vi "map_trap_switch_stiffback.vi"() -> ()   [LabVIEW 2015]
panel:
  out "Mapping file":string
  in  "Done ?":bool
  in  "KILL":bool
  in  "PAUSE":bool
  in  "RESUME":bool
  in  "QUIT":bool
  in  "up done":bool
  in  "z up":bool
  in  "Done":bool
  in  "z piastra":bool
  in  "x piastra":bool
  in  "goto y pos":bool
  in  "goto x pos":bool
  in  "End":bool
  in  "zero z - end":bool
  in  "zero x - end":bool
  in  "zero y - end":bool
  in  "positioning done":bool
  out "output":string
  out "command":string
  in  "zero done":bool
  in  "zero z":bool
  in  "zero x":bool
  in  "zero y":bool
  # "Comandi di emergenza"
  # "Posiziono in zero"
  # "Vado sulla piastra \ne azzero"
  # "Alzo il laser"
  # "Vado in posizione"
  # "Ritorno a zero"
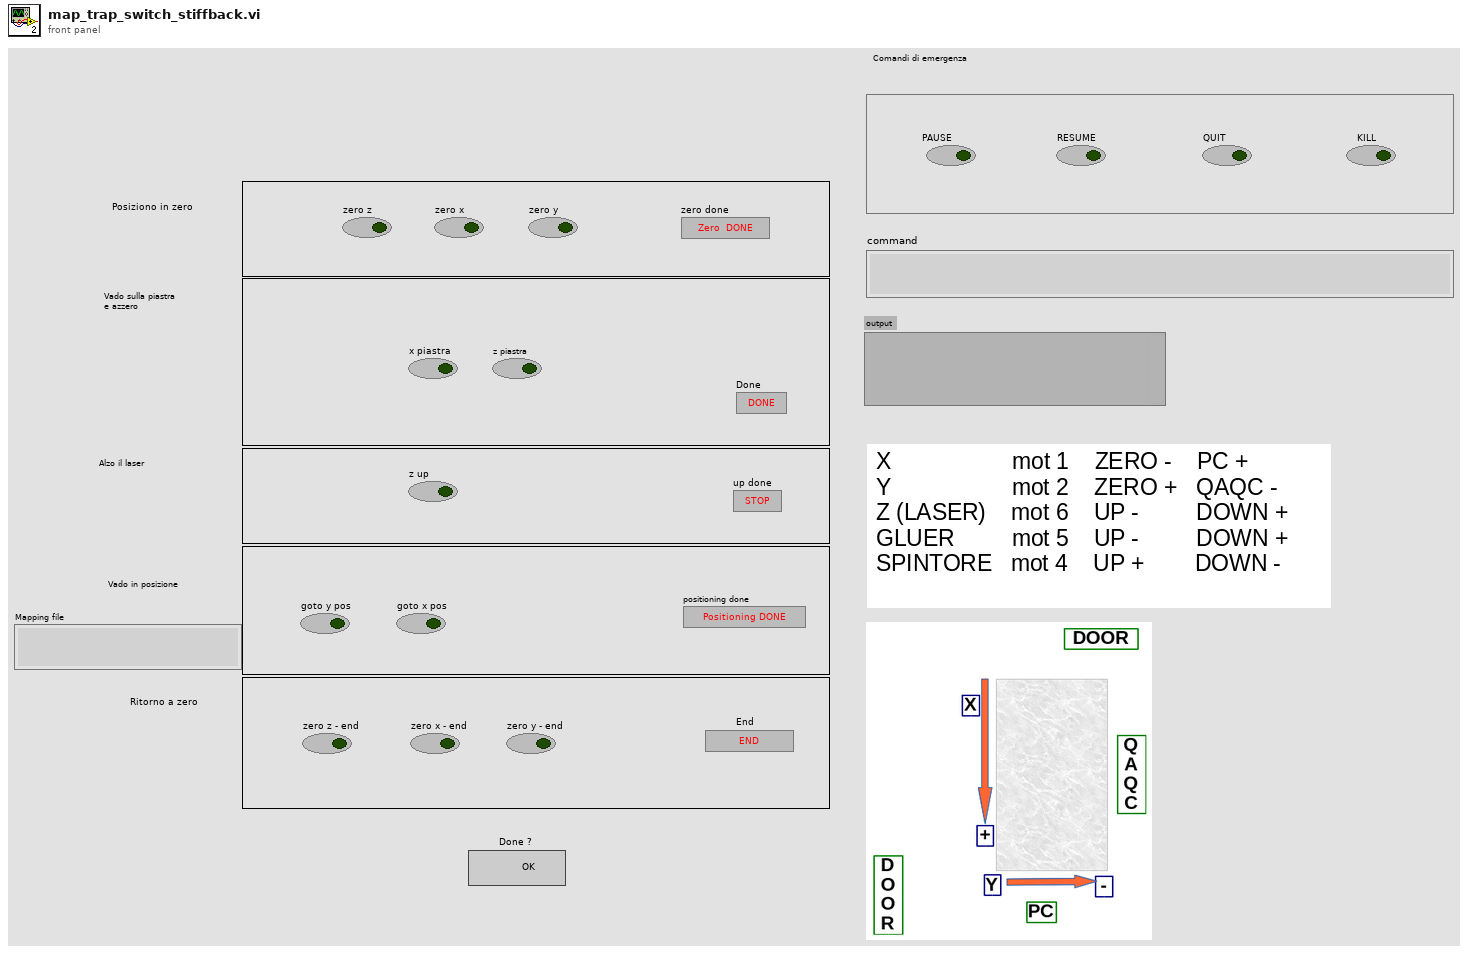
[diagram p1: front panel]
types:
  T1 = enum16{"open", "replace", "create", "open or create", "replace or create", "replace or create with confirmation"}
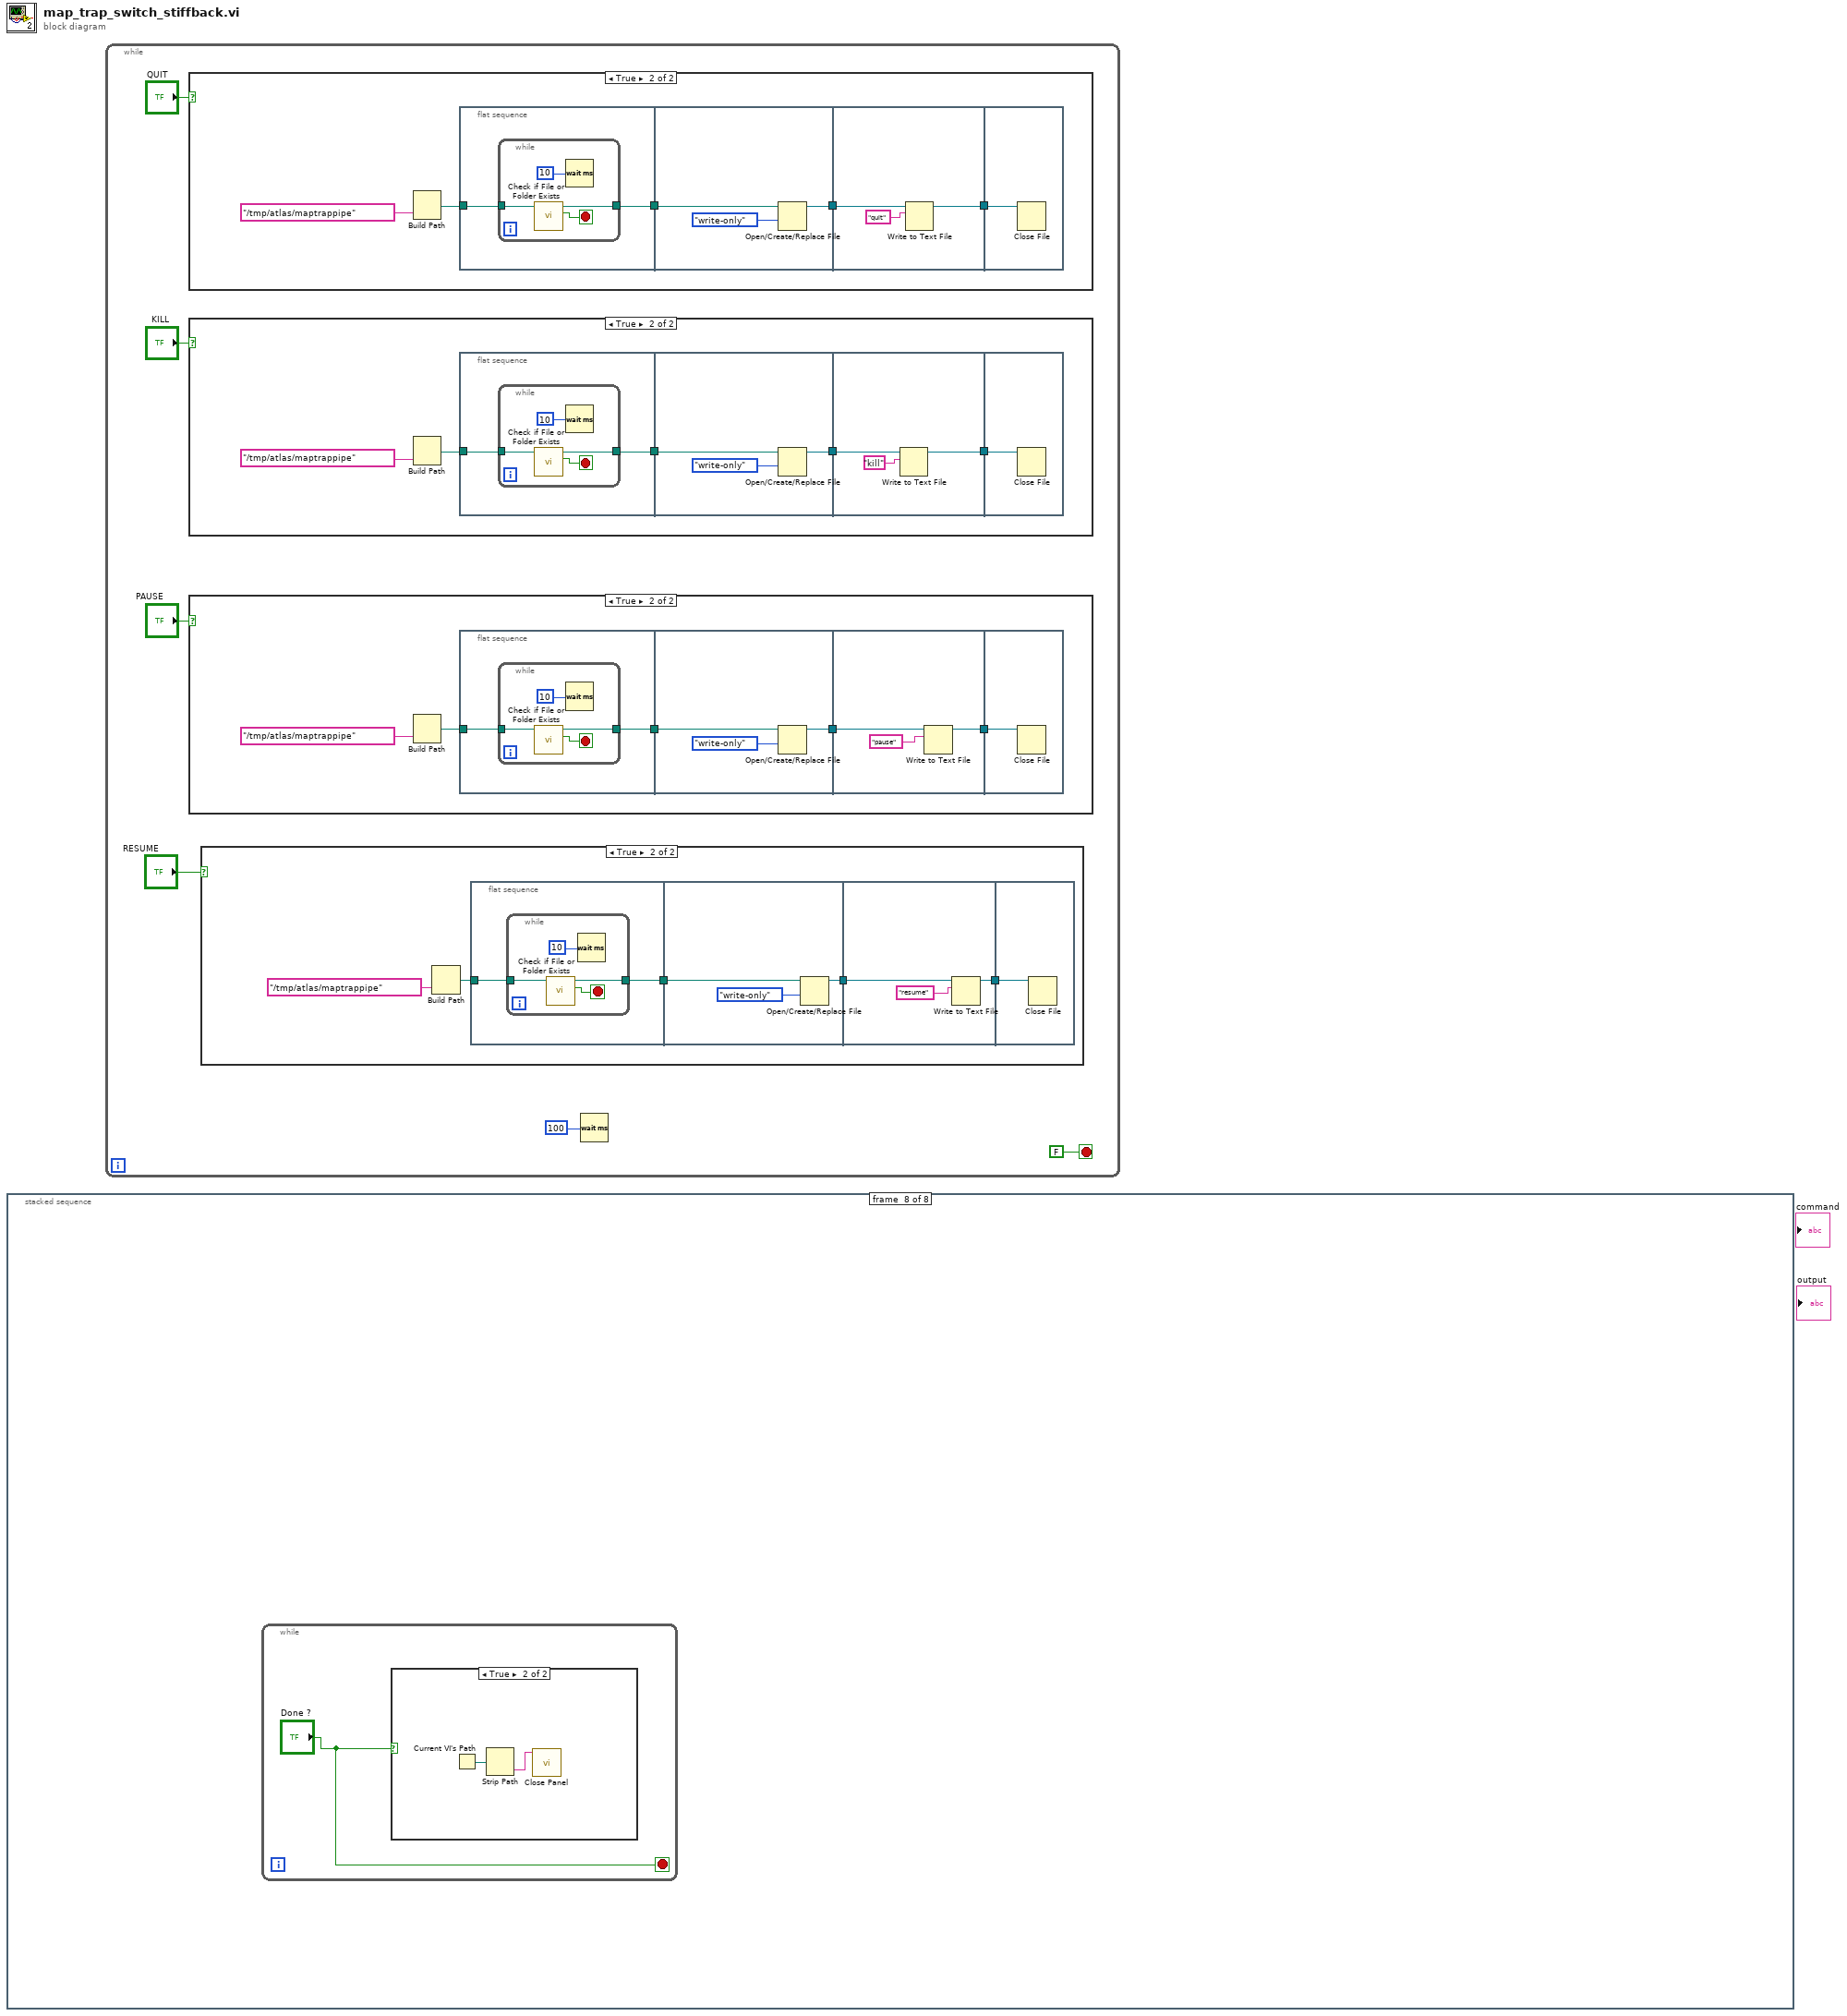
[diagram p0: block diagram]
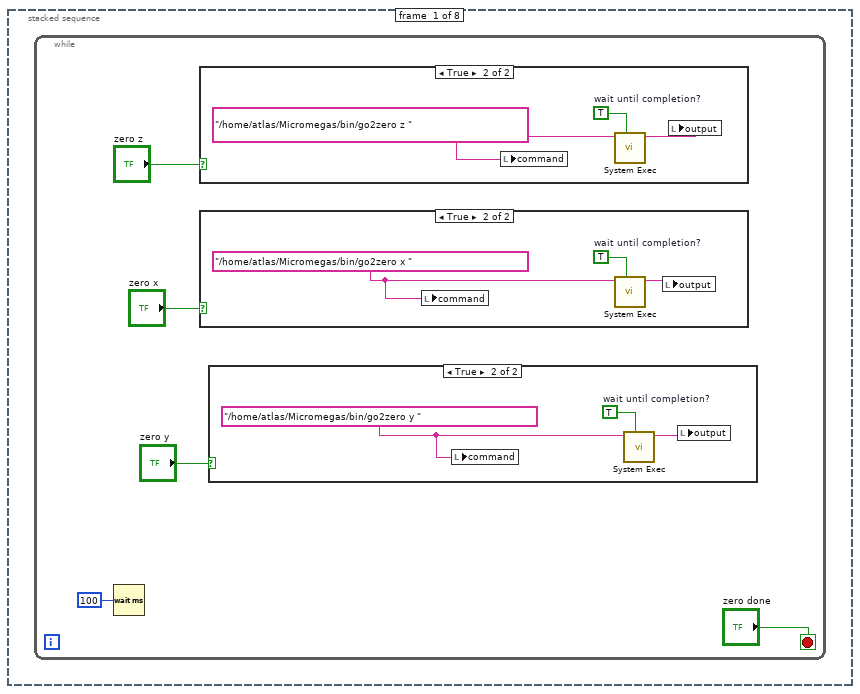
[diagram p6: hidden frame]
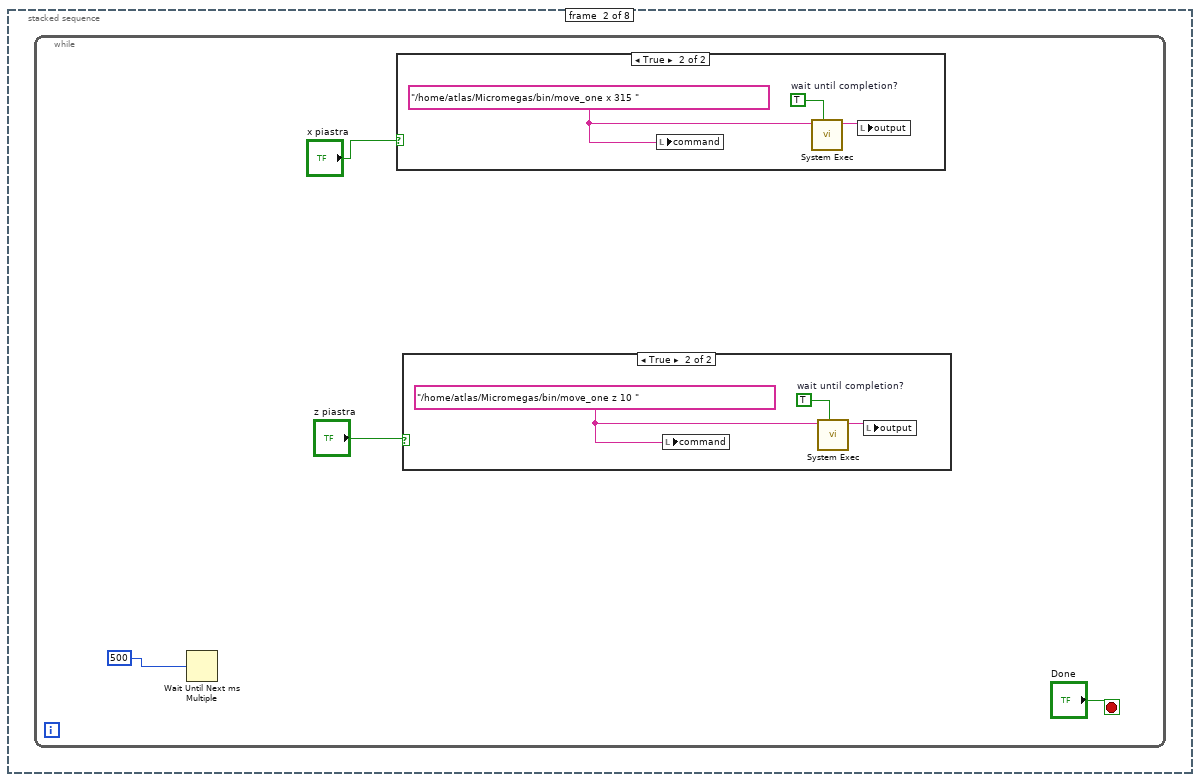
[diagram p10: hidden frame]
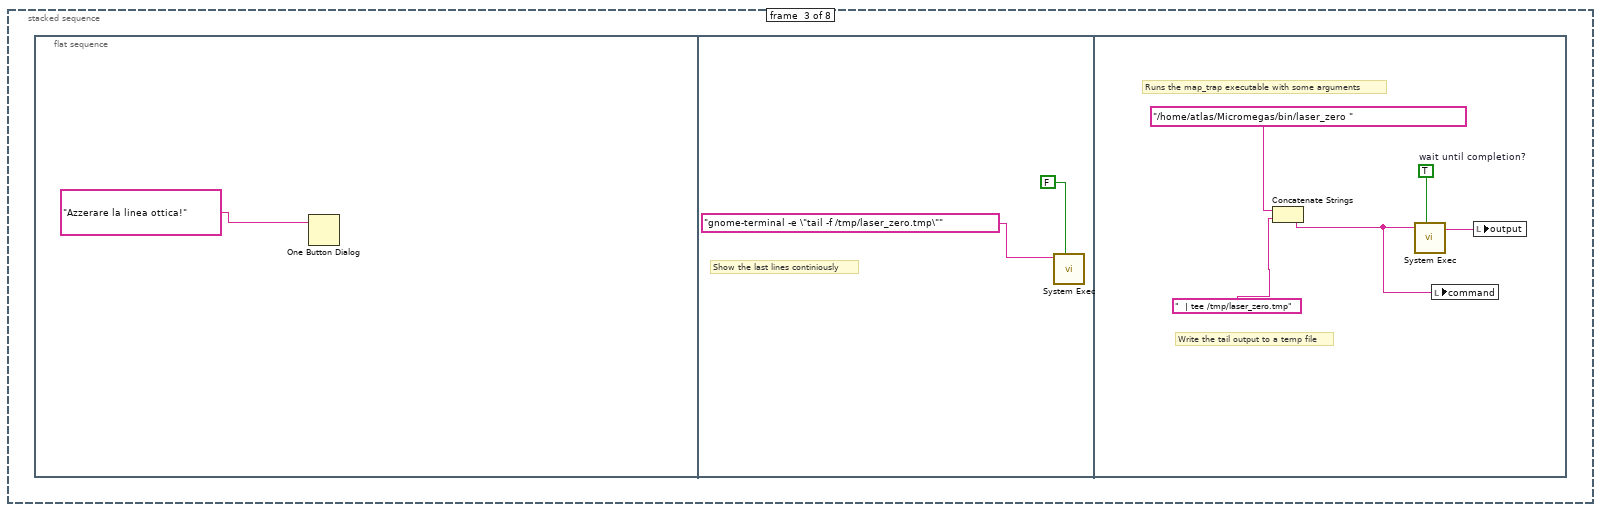
[diagram p13: hidden frame]
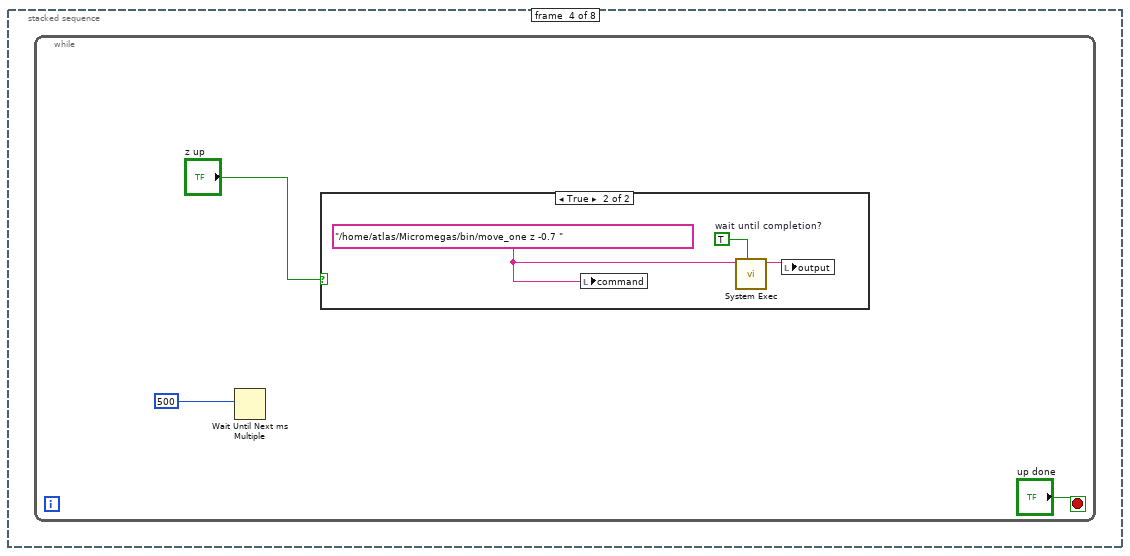
[diagram p14: hidden frame]
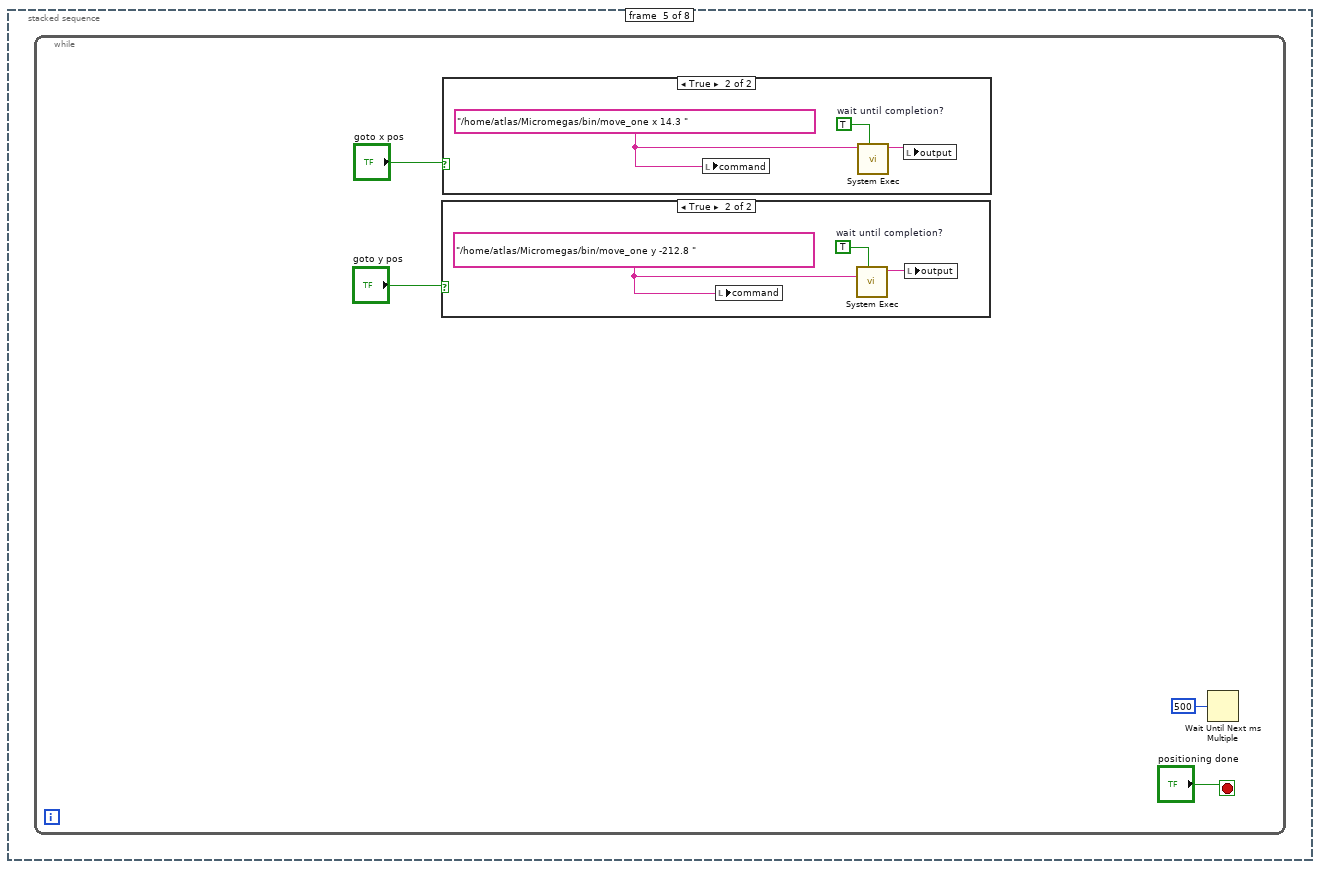
[diagram p16: hidden frame]
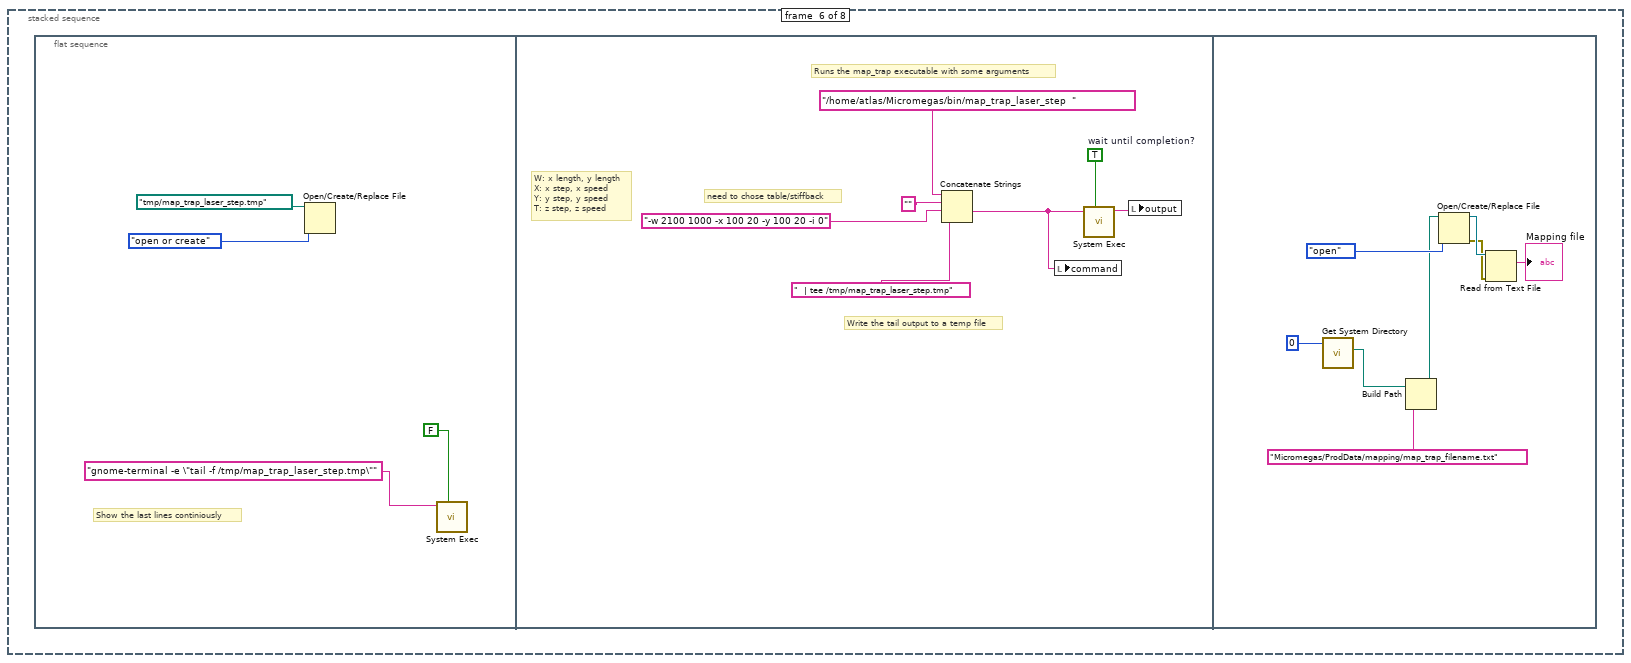
[diagram p19: hidden frame]
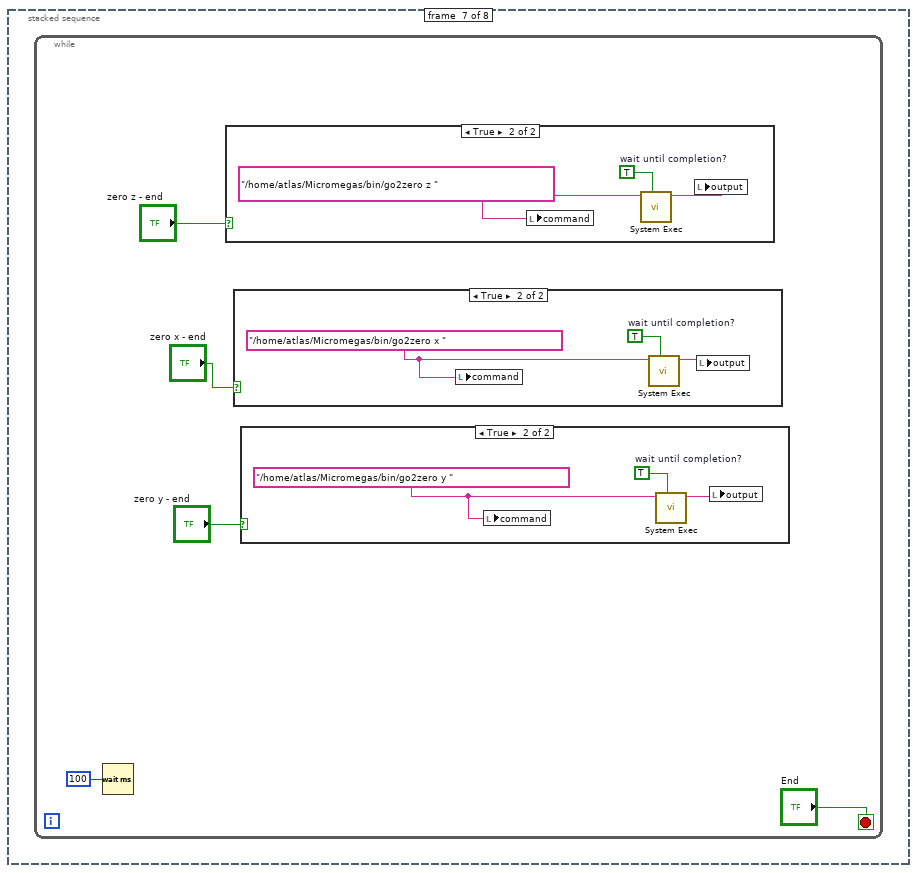
[diagram p20: hidden frame]
diagram:
  n1 = stacked-sequence {
    frame #0 {
      n2 = while {
        stop <- "zero done" stop-if-true
        n3 = Wait (ms)(milliseconds to wait=u32 100) -> ()  [unwired: 1 out]
        n4 = case shown="True" "zero z" {
          frame False {
          }
          frame True {
            w13 = "/home/atlas/Micromegas/bin/go2zero z " ("string")
            w14 = TRUE  # wait until completion?
            n5 = local write "command"(w13) -> ()
            n6 = call <vilib>:"System Exec.vi"("wait until completion? (T)"=w14, "command line"=w13) -> ("standard output"=w12:string)  [unwired: 6 in, 3 out]
            n7 = local write "output"(w12) -> ()
          }
        }
        n8 = case shown="True" "zero x" {
          frame False {
          }
          frame True {
            w10 = "/home/atlas/Micromegas/bin/go2zero x " ("string")
            w11 = TRUE  # wait until completion?
            n9 = local write "command"(w10) -> ()
            n10 = call <vilib>:"System Exec.vi"("wait until completion? (T)"=w11, "command line"=w10) -> ("standard output"=w9:string)  [unwired: 6 in, 3 out]
            n11 = local write "output"(w9) -> ()
          }
        }
        n12 = case shown="True" "zero y" {
          frame False {
          }
          frame True {
            w7 = "/home/atlas/Micromegas/bin/go2zero y " ("string")
            w8 = TRUE  # wait until completion?
            n13 = local write "command"(w7) -> ()
            n14 = call <vilib>:"System Exec.vi"("wait until completion? (T)"=w8, "command line"=w7) -> ("standard output"=w6:string)  [unwired: 6 in, 3 out]
            n15 = local write "output"(w6) -> ()
          }
        }
      }
    }
    frame #1 {
      n16 = while {
        stop <- "Done" stop-if-true
        n17 = Wait Until Next ms Multiple(millisecond multiple=u32 500 ("millisecond timer value")) -> ()  [unwired: 1 out]
        n18 = case shown="True" "x piastra" {
          frame False {
          }
          frame True {
            w22 = "/home/atlas/Micromegas/bin/move_one x 315 " ("string")
            w24 = TRUE  # wait until completion?
            n19 = local write "command"(w22) -> ()
            n20 = call <vilib>:"System Exec.vi"("wait until completion? (T)"=w24, "command line"=w22) -> ("standard output"=w23:string)  [unwired: 6 in, 3 out]
            n21 = local write "output"(w23) -> ()
          }
        }
        n22 = case shown="True" "z piastra" {
          frame False {
          }
          frame True {
            w19 = "/home/atlas/Micromegas/bin/move_one z 10 " ("string")
            w21 = TRUE  # wait until completion?
            n23 = local write "command"(w19) -> ()
            n24 = call <vilib>:"System Exec.vi"("wait until completion? (T)"=w21, "command line"=w19) -> ("standard output"=w20:string)  [unwired: 6 in, 3 out]
            n25 = local write "output"(w20) -> ()
          }
        }
      }
    }
    frame #2 {
      n26 = flat-sequence {
        frame #0 {
          n27 = One Button Dialog(message="Azzerare la linea ottica!") -> ()  [unwired: 1 in, 1 out]
        }
        frame #1 {
          # "Show the last lines continiously"
          n28 = call <vilib>:"System Exec.vi"("wait until completion? (T)"=FALSE, "command line"="gnome-terminal -e \"tail -f /tmp/laser_zero.tmp\"") -> ()  [unwired: 6 in, 4 out]
        }
        frame #2 {
          w32 = TRUE  # wait until completion?
          # "Write the tail output to a temp file"
          # "Runs the map_trap executable with some arguments"
          n29 = Concatenate Strings("/home/atlas/Micromegas/bin/laser_zero " ("string"), "  | tee /tmp/laser_zero.tmp" ("string")) -> (w28:string)
          n30 = call <vilib>:"System Exec.vi"("wait until completion? (T)"=w32, "command line"=w28) -> ("standard output"=w29:string)  [unwired: 6 in, 3 out]
          n31 = local write "command"(w28) -> ()
          n32 = local write "output"(w29) -> ()
        }
      }
    }
    frame #3 {
      n33 = while {
        stop <- "up done" stop-if-true
        n34 = Wait Until Next ms Multiple(millisecond multiple=u32 500 ("millisecond timer value")) -> ()  [unwired: 1 out]
        n35 = case shown="True" "z up" {
          frame False {
          }
          frame True {
            w36 = "/home/atlas/Micromegas/bin/move_one z -0.7 " ("string")
            w38 = TRUE  # wait until completion?
            n36 = local write "command"(w36) -> ()
            n37 = call <vilib>:"System Exec.vi"("wait until completion? (T)"=w38, "command line"=w36) -> ("standard output"=w37:string)  [unwired: 6 in, 3 out]
            n38 = local write "output"(w37) -> ()
          }
        }
      }
    }
    frame #4 {
      n39 = while {
        stop <- "positioning done" stop-if-true
        n40 = case shown="True" "goto y pos" {
          frame False {
          }
          frame True {
            w43 = "/home/atlas/Micromegas/bin/move_one y -212.8 " ("string")
            w45 = TRUE  # wait until completion?
            n41 = local write "command"(w43) -> ()
            n42 = call <vilib>:"System Exec.vi"("wait until completion? (T)"=w45, "command line"=w43) -> ("standard output"=w44:string)  [unwired: 6 in, 3 out]
            n43 = local write "output"(w44) -> ()
          }
        }
        n44 = case shown="True" "goto x pos" {
          frame False {
          }
          frame True {
            w46 = "/home/atlas/Micromegas/bin/move_one x 14.3 " ("string")
            w48 = TRUE  # wait until completion?
            n45 = local write "command"(w46) -> ()
            n46 = call <vilib>:"System Exec.vi"("wait until completion? (T)"=w48, "command line"=w46) -> ("standard output"=w47:string)  [unwired: 6 in, 3 out]
            n47 = local write "output"(w47) -> ()
          }
        }
        n48 = Wait Until Next ms Multiple(millisecond multiple=u32 500) -> ()  [unwired: 1 out]
      }
    }
    frame #5 {
      n49 = flat-sequence {
        frame #0 {
          # "Show the last lines continiously"
          n50 = Open/Create/Replace File(file path (use dialog)=path "/tmp/map_trap_laser_step.tmp", operation (0:open)=T1."open or create") -> ()  [unwired: 4 in, 3 out]
          n51 = call <vilib>:"System Exec.vi"("wait until completion? (T)"=FALSE, "command line"="gnome-terminal -e \"tail -f /tmp/map_trap_laser_step.tmp\"") -> ()  [unwired: 6 in, 4 out]
        }
        frame #1 {
          w59 = TRUE  # wait until completion?
          # "need to chose table/stiffback"
          # "Write the tail output to a temp file"
          # "Runs the map_trap executable with some arguments"
          # "W: x length, y length\nX: x step, x speed\nY: y step, y speed\nT: z step, z speed"
          n52 = Concatenate Strings("/home/atlas/Micromegas/bin/map_trap_laser_step  " ("string"), "" ("string"), "-w 2100 1000 -x 100 20 -y 100 20 -i 0" ("string"), "  | tee /tmp/map_trap_laser_step.tmp" ("string")) -> (w54:string)
          n53 = local write "command"(w54) -> ()
          n54 = call <vilib>:"System Exec.vi"("wait until completion? (T)"=w59, "command line"=w54) -> ("standard output"=w53:string)  [unwired: 6 in, 3 out]
          n55 = local write "output"(w53) -> ()
        }
        frame #2 {
          n56 = call <vilib>:"Get System Directory.vi"("system directory type"=0) -> ("system directory"=w61:path)  [unwired: 10 in]
          n57 = Build Path(base path=w61, name or relative path="Micromegas/ProdData/mapping/map_trap_filename.txt") -> (appended path=w60:path)
          n58 = Open/Create/Replace File(file path (use dialog)=w60, operation (0:open)=T1."open") -> (refnum out=w66:refnum<file>, error out=w65:errorcluster)  [unwired: 4 in, 1 out]
          n59 = Read from Text File(file (use dialog)=w66, error in=w65) -> (text=→"Mapping file":string)  [unwired: 2 in, 3 out]
        }
      }
    }
    frame #6 {
      n60 = while {
        stop <- "End" stop-if-true
        n61 = Wait (ms)(milliseconds to wait=u32 100) -> ()  [unwired: 1 out]
        n62 = case shown="True" "zero z - end" {
          frame False {
          }
          frame True {
            w80 = "/home/atlas/Micromegas/bin/go2zero z " ("string")
            w81 = TRUE  # wait until completion?
            n63 = local write "command"(w80) -> ()
            n64 = call <vilib>:"System Exec.vi"("wait until completion? (T)"=w81, "command line"=w80) -> ("standard output"=w79:string)  [unwired: 6 in, 3 out]
            n65 = local write "output"(w79) -> ()
          }
        }
        n66 = case shown="True" "zero x - end" {
          frame False {
          }
          frame True {
            w77 = "/home/atlas/Micromegas/bin/go2zero x " ("string")
            w78 = TRUE  # wait until completion?
            n67 = local write "command"(w77) -> ()
            n68 = call <vilib>:"System Exec.vi"("wait until completion? (T)"=w78, "command line"=w77) -> ("standard output"=w76:string)  [unwired: 6 in, 3 out]
            n69 = local write "output"(w76) -> ()
          }
        }
        n70 = case shown="True" "zero y - end" {
          frame False {
          }
          frame True {
            w74 = "/home/atlas/Micromegas/bin/go2zero y " ("string")
            w75 = TRUE  # wait until completion?
            n71 = local write "command"(w74) -> ()
            n72 = call <vilib>:"System Exec.vi"("wait until completion? (T)"=w75, "command line"=w74) -> ("standard output"=w73:string)  [unwired: 6 in, 3 out]
            n73 = local write "output"(w73) -> ()
          }
        }
      }
    }
    frame #7 {
      n74 = while {
        stop <- "Done ?" stop-if-true
        n75 = case shown="True" "Done ?" {
          frame False {
          }
          frame True {
            n76 = Current VI's Path() -> (path=w83:path)
            n77 = Strip Path(path=w83) -> (name=w84:string)  [unwired: 1 out]
            n78 = call <vilib>:"Close Panel.vi"("VI name"=w84) -> ()  [unwired: 10 in, 1 out]
          }
        }
      }
    }
  }
  n79 = while {
    stop <- FALSE stop-if-true
    n80 = case shown="True" "QUIT" {
      frame False {
      }
      frame True {
        n81 = Build Path(name or relative path="/tmp/atlas/maptrappipe" ("string")) -> (appended path=w145:path)  [unwired: 1 in]
        n82 = flat-sequence {
          tunnel: [w151] -> w149
          tunnel: w145 -> [w150]
          tunnel: w149 -> [w158]
          tunnel: [w156] -> w148
          tunnel: w148 -> [w161]
          tunnel: [w160] -> w147
          tunnel: w147 -> [w162]
          frame #0 {
            n83 = while {
              tunnel: [w153] -> w151
              tunnel: w150 -> [w152]
              stop <- w154 stop-if-true
              n84 = call <vilib>:"Check if File or Folder Exists.vi"("path"=w152) -> ("file or folder exists?"=w154:bool, "dup path"=w153:path)  [unwired: 8 in, 1 out]
              n85 = Wait (ms)(milliseconds to wait=u32 10) -> ()  [unwired: 1 out]
            }
          }
          frame #1 {
            n86 = Open/Create/Replace File(file path (use dialog)=w158, access (0:read/write)=enum16{"read/write", "read-only", "write-only"}."write-only") -> (refnum out=w156:refnum<file>)  [unwired: 4 in, 2 out]
          }
          frame #2 {
            n87 = Write to Text File(file (use dialog)=w161, text="quit") -> (refnum out=w160:refnum<file>)  [unwired: 2 in, 2 out]
          }
          frame #3 {
            n88 = Close File(refnum=w162) -> ()  [unwired: 1 in, 2 out]
          }
        }
      }
    }
    n89 = case shown="True" "KILL" {
      frame False {
      }
      frame True {
        n90 = Build Path(name or relative path="/tmp/atlas/maptrappipe" ("string")) -> (appended path=w109:path)  [unwired: 1 in]
        n91 = flat-sequence {
          tunnel: [w115] -> w113
          tunnel: w109 -> [w114]
          tunnel: w113 -> [w122]
          tunnel: [w120] -> w112
          tunnel: w112 -> [w125]
          tunnel: [w124] -> w111
          tunnel: w111 -> [w126]
          frame #0 {
            n92 = while {
              tunnel: [w117] -> w115
              tunnel: w114 -> [w116]
              stop <- w118 stop-if-true
              n93 = call <vilib>:"Check if File or Folder Exists.vi"("path"=w116) -> ("file or folder exists?"=w118:bool, "dup path"=w117:path)  [unwired: 8 in, 1 out]
              n94 = Wait (ms)(milliseconds to wait=u32 10) -> ()  [unwired: 1 out]
            }
          }
          frame #1 {
            n95 = Open/Create/Replace File(file path (use dialog)=w122, access (0:read/write)=enum16{"read/write", "read-only", "write-only"}."write-only") -> (refnum out=w120:refnum<file>)  [unwired: 4 in, 2 out]
          }
          frame #2 {
            n96 = Write to Text File(file (use dialog)=w125, text="kill") -> (refnum out=w124:refnum<file>)  [unwired: 2 in, 2 out]
          }
          frame #3 {
            n97 = Close File(refnum=w126) -> ()  [unwired: 1 in, 2 out]
          }
        }
      }
    }
    n98 = case shown="True" "PAUSE" {
      frame False {
      }
      frame True {
        n99 = Build Path(name or relative path="/tmp/atlas/maptrappipe" ("string")) -> (appended path=w91:path)  [unwired: 1 in]
        n100 = flat-sequence {
          tunnel: [w97] -> w95
          tunnel: w91 -> [w96]
          tunnel: w95 -> [w104]
          tunnel: [w102] -> w94
          tunnel: w94 -> [w107]
          tunnel: [w106] -> w93
          tunnel: w93 -> [w108]
          frame #0 {
            n101 = while {
              tunnel: [w99] -> w97
              tunnel: w96 -> [w98]
              stop <- w100 stop-if-true
              n102 = call <vilib>:"Check if File or Folder Exists.vi"("path"=w98) -> ("file or folder exists?"=w100:bool, "dup path"=w99:path)  [unwired: 8 in, 1 out]
              n103 = Wait (ms)(milliseconds to wait=u32 10) -> ()  [unwired: 1 out]
            }
          }
          frame #1 {
            n104 = Open/Create/Replace File(file path (use dialog)=w104, access (0:read/write)=enum16{"read/write", "read-only", "write-only"}."write-only") -> (refnum out=w102:refnum<file>)  [unwired: 4 in, 2 out]
          }
          frame #2 {
            n105 = Write to Text File(file (use dialog)=w107, text="pause") -> (refnum out=w106:refnum<file>)  [unwired: 2 in, 2 out]
          }
          frame #3 {
            n106 = Close File(refnum=w108) -> ()  [unwired: 1 in, 2 out]
          }
        }
      }
    }
    n107 = case shown="True" "RESUME" {
      frame False {
      }
      frame True {
        n108 = Build Path(name or relative path="/tmp/atlas/maptrappipe" ("string")) -> (appended path=w127:path)  [unwired: 1 in]
        n109 = flat-sequence {
          tunnel: [w133] -> w131
          tunnel: w127 -> [w132]
          tunnel: w131 -> [w140]
          tunnel: [w138] -> w130
          tunnel: w130 -> [w143]
          tunnel: [w142] -> w129
          tunnel: w129 -> [w144]
          frame #0 {
            n110 = while {
              tunnel: [w135] -> w133
              tunnel: w132 -> [w134]
              stop <- w136 stop-if-true
              n111 = call <vilib>:"Check if File or Folder Exists.vi"("path"=w134) -> ("file or folder exists?"=w136:bool, "dup path"=w135:path)  [unwired: 8 in, 1 out]
              n112 = Wait (ms)(milliseconds to wait=u32 10) -> ()  [unwired: 1 out]
            }
          }
          frame #1 {
            n113 = Open/Create/Replace File(file path (use dialog)=w140, access (0:read/write)=enum16{"read/write", "read-only", "write-only"}."write-only") -> (refnum out=w138:refnum<file>)  [unwired: 4 in, 2 out]
          }
          frame #2 {
            n114 = Write to Text File(file (use dialog)=w143, text="resume") -> (refnum out=w142:refnum<file>)  [unwired: 2 in, 2 out]
          }
          frame #3 {
            n115 = Close File(refnum=w144) -> ()  [unwired: 1 in, 2 out]
          }
        }
      }
    }
    n116 = Wait (ms)(milliseconds to wait=100) -> ()  [unwired: 1 out]
  }
